vi "Ultrasonic.vi"(1 "State Control":enum16{"Open", "Run", "End"}(ring)) -> (0 "Distance (in.)":dbl)   [LabVIEW 2013]
uses:
  <vilib>/Rock Robotics/SystemInterfaces/AI/FPGA_AIChannel.ctl
panel:
  in  "Right":T1=enum."AI 2"
  in  "Scaling factor (V/in)":dbl=0.0098
  in  "Average Bits":u8=6
  in  "Samples Per Second":dbl=1000.0
  out "Distance (in.)":dbl(slide)=125.0 scale=0.0..250.0 scale format="%3d"
  out "Waveform Chart":dbl(graph)
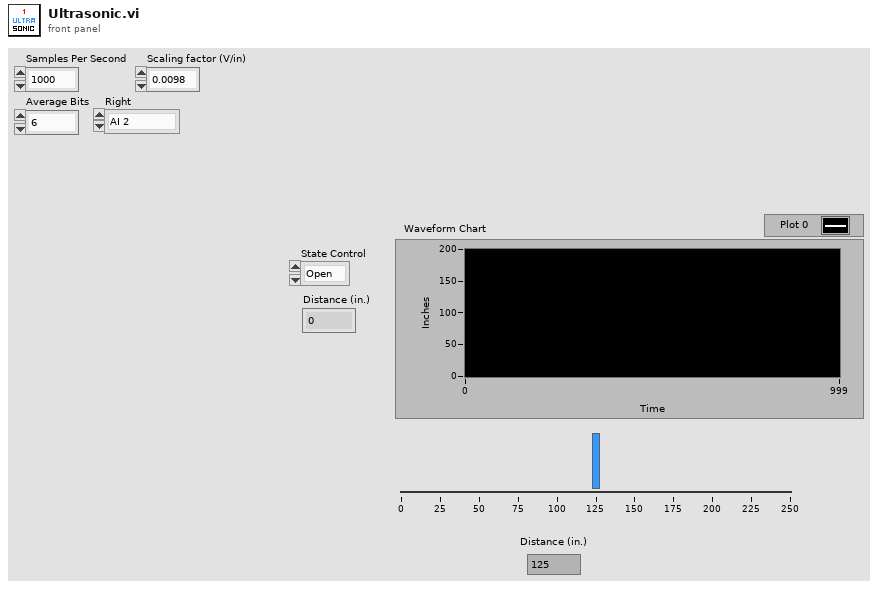
[diagram p1: front panel]
types:
  T1 = typedef "FPGA_AIChannel.ctl" = enum8{"AI 1", "AI 2", "AI 3", "AI 4", "AI 5", "AI 6", "AI 7", "AI 8", "Invalid"}
  T2 = typedef "WPI_AnalogChannelDevRef.ctl" = cluster{"DevStatus":errorcluster, "Analog Module":T3, "Analog Channel":T1}
  T3 = typedef "FPGA_TypedefAnalogModule.ctl" = enum16{"Analog Module 1", "Analog Module 2"}
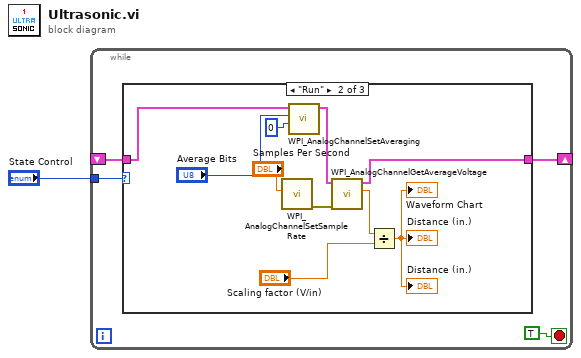
[diagram p0: block diagram]
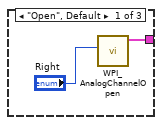
[diagram p2: hidden frame]
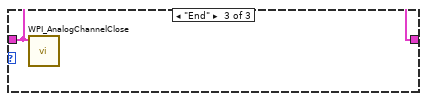
[diagram p3: hidden frame]
diagram:
  n1 = while {
    tunnel: "State Control" -> [w5]
    shift-right: [w4] -> _
    shift-left: _ -> [w3]
    stop <- TRUE stop-if-true
    n2 = case shown="\"Run\"" w5 {
      tunnel: [w6 w9 w18] -> w4
      tunnel: w3 -> [_ w10 w18]
      frame "Open", Default {
        n3 = call <vilib>:"WPI_AnalogChannelOpen.vi"("Analog Channel"="Right") -> ("AIDeviceRef"=w6:T2)  [unwired: 2 in, 8 out]
      }
      frame "Run" {
        n4 = call <vilib>:"WPI_AnalogChannelSetSampleRate.vi"("Samples Per Second"="Samples Per Second") -> ("error out"=w11:errorcluster)  [unwired: 3 in, 7 out]
        n5 = call <vilib>:"WPI_AnalogChannelSetAveraging.vi"("OversampleBits"=u8 0, "AverageBits"="Average Bits", "AIDeviceRef"=w10) -> ("AIDeviceRef"=w12:T2)  [unwired: 1 in, 7 out]
        n6 = call <vilib>:"WPI_AnalogChannelGetAverageVoltage.vi"("error in (no error)"=w11, "AIDeviceRef"=w12) -> ("Voltage"=w13:dbl, "AIDeviceRef"=w9:T2)  [unwired: 8 out]
        n7 = Divide(x=w13, y="Scaling factor (V/in)") -> (x/y=→"Distance (in.)" →"Waveform Chart" →"Distance (in.)":dbl)
      }
      frame "End" {
        n8 = call <vilib>:"WPI_AnalogChannelClose.vi"("AIDeviceRef"=w18) -> ()  [unwired: 1 in, 10 out]
      }
    }
  }
